vi "Construct Reader.vi"(11 "Reader Enum in":T1=enum."Cryostat Temperature") -> (0 "error out":errorcluster, 3 "Reader out":refnum<class "Reader.lvclass">)   [LabVIEW 2017, in "Scan Driver.lvclass"]
uses:
  Scan Driver.lvclass
  Reader List.ctl
  Readers/Reader/Reader.lvclass
  Readers/PC Reader/PC Reader.lvclass
  C:/LabVIEW-programs/Readers/Reader/Reader.lvclass
  Instruments/Lockin/Lockin SR830.lvclass
  C:/LabVIEW-programs/Instruments/Utility Classes/Readable/Readable.lvclass
  Instruments/Utility Classes/Dummy/Dummy.lvclass
  Instruments/DAQ/DAQmx Analog.lvclass
  Instruments/Oxford Magnet/Temperature Controller/Temperature Controller.lvclass
  Instruments/Fluke Multimeter/Fluke Multimeter.lvclass
  Instruments/Power Meter/Power Meter.lvclass
  Instruments/Cryostat/Cryostat.lvclass
  Instruments/Photon Counter/Photon Counter SR400.lvclass
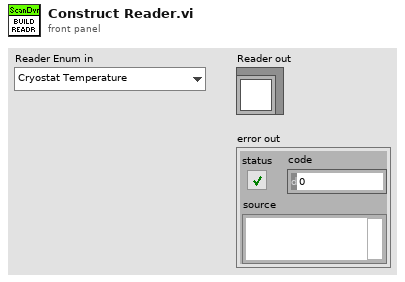
[diagram p1: front panel]
types:
  T1 = typedef "Scan Driver.lvclass/Reader List.ctl" = enum16{"Dummy", "Cryostat Temperature", "DAQmx Analog", "Lockin SR830", "Multimeter", "Photon Counter", "Power Meter", "Temperature Control"}
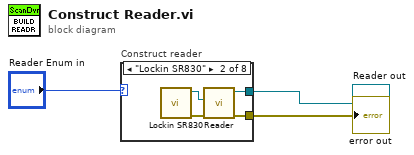
[diagram p0: block diagram]
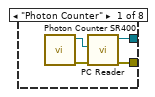
[diagram p2: hidden frame]
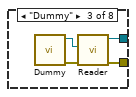
[diagram p3: hidden frame]
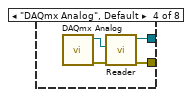
[diagram p4: hidden frame]
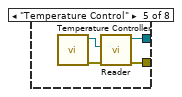
[diagram p5: hidden frame]
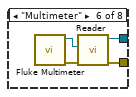
[diagram p6: hidden frame]
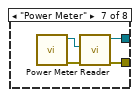
[diagram p7: hidden frame]
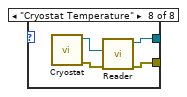
[diagram p8: hidden frame]
diagram:
  n1 = case "Construct reader" shown="\"Lockin SR830\"" "Reader Enum in" {
    tunnel: [w6 w10 w14 w18 w23 w25 w29 w33] -> w1
    tunnel: [w4 w8 w12 w16 w22 w24 w28 w32] -> w2
    frame "Photon Counter" {
      n2 = call "Photon Counter SR400.vi"() -> ("error out"=w5:errorcluster, "Photon Counter SR400 out"=w7:refnum<class "Photon Counter SR400.lvclass">)  [unwired: 10 out]
      n3 = call "PC Reader.vi"("error in (no error)"=w5, "Photon Counter SR400 in"=w7) -> ("error out"=w4:errorcluster, "PC Reader out"=w6:refnum<class "PC Reader.lvclass">)  [unwired: 8 out]
    }
    frame "Lockin SR830" {
      n4 = call "Lockin SR830.vi"() -> ("error out"=w9:errorcluster, "Lockin SR830 out"=w11:refnum<class "Lockin SR830.lvclass">)  [unwired: 1 in, 9 out]
      n5 = call "Reader.vi"("error in (no error)"=w9, "Readable"=w11) -> ("error out"=w8:errorcluster, "Reader out"=w10:refnum<class "Reader.lvclass">)  [unwired: 8 out]
    }
    frame "Dummy" {
      n6 = call "Dummy.vi"() -> ("error out"=w13:errorcluster, "Dummy out"=w15:refnum<class "Dummy.lvclass">)  [unwired: 2 in, 8 out]
      n7 = call "Reader.vi"("error in (no error)"=w13, "Readable"=w15) -> ("error out"=w12:errorcluster, "Reader out"=w14:refnum<class "Reader.lvclass">)  [unwired: 8 out]
    }
    frame "DAQmx Analog", Default {
      n8 = call "DAQmx Analog.vi"() -> ("error out"=w17:errorcluster, "DAQmx Analog out"=w19:refnum<class "DAQmx Analog.lvclass">)  [unwired: 1 in, 9 out]
      n9 = call "Reader.vi"("error in (no error)"=w17, "Readable"=w19) -> ("error out"=w16:errorcluster, "Reader out"=w18:refnum<class "Reader.lvclass">)  [unwired: 8 out]
    }
    frame "Temperature Control" {
      n10 = call "Temperature Controller.vi"() -> ("error out"=w21:errorcluster, "Temperature Controller out"=w20:refnum<class "Temperature Controller.lvclass">)  [unwired: 10 in]
      n11 = call "Reader.vi"("error in (no error)"=w21, "Readable"=w20) -> ("error out"=w22:errorcluster, "Reader out"=w23:refnum<class "Reader.lvclass">)  [unwired: 8 out]
    }
    frame "Multimeter" {
      n12 = call "Fluke Multimeter.vi"() -> ("error out"=w27:errorcluster, "Fluke Multimeter out"=w26:refnum<class "Fluke Multimeter.lvclass">)  [unwired: 10 in]
      n13 = call "Reader.vi"("error in (no error)"=w27, "Readable"=w26) -> ("error out"=w24:errorcluster, "Reader out"=w25:refnum<class "Reader.lvclass">)  [unwired: 8 out]
    }
    frame "Power Meter" {
      n14 = call "Power Meter.vi"() -> ("error out"=w31:errorcluster, "Power Meter out"=w30:refnum<class "Power Meter.lvclass">)  [unwired: 10 in]
      n15 = call "Reader.vi"("error in (no error)"=w31, "Readable"=w30) -> ("error out"=w28:errorcluster, "Reader out"=w29:refnum<class "Reader.lvclass">)  [unwired: 8 out]
    }
    frame "Cryostat Temperature" {
      n16 = call "Cryostat.vi"() -> ("error out"=w34:errorcluster, "Cryostat out"=w35:refnum<class "Cryostat.lvclass">)  [unwired: 10 in]
      n17 = call "Reader.vi"("error in (no error)"=w34, "Readable"=w35) -> ("error out"=w32:errorcluster, "Reader out"=w33:refnum<class "Reader.lvclass">)  [unwired: 8 out]
    }
  }
  "error out" <- w2
  "Reader out" <- w1
